vi "Set New Value Blue Pixel.vi"(8 "Bit to code":u8, 9 "Energy":dbl, 10 "General Brightness":dbl, 11 "B":u8) -> (3 "New B value Out":u8)   [LabVIEW 2015]
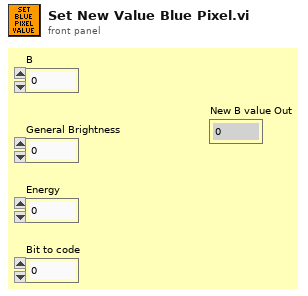
[diagram p1: front panel]
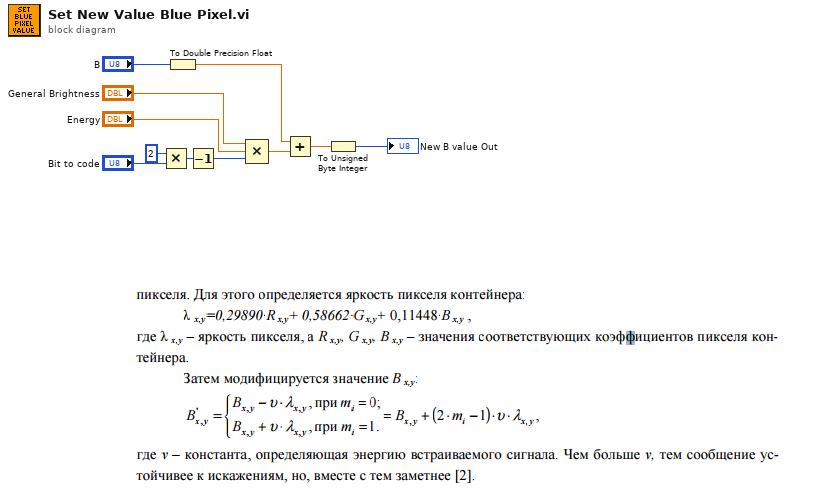
[diagram p0: block diagram]
diagram:
  n1 = Multiply(x=u8 2, y="Bit to code") -> (x*y=w9:u8)
  n2 = To Double Precision Float(number="B") -> (double precision float=w2:dbl)
  n3 = Decrement(x=w9) -> (x-1=w8:u8)
  n4 = Compound Arithmetic op=MULTIPLY("General Brightness", "Energy", w8) -> (w5:dbl)
  n5 = Add(x=w2, y=w5) -> (x+y=w3:dbl)
  n6 = To Unsigned Byte Integer(number=w3) -> (unsigned 8bit integer=→"New B value Out":u8)
